vi "Comments.Add Wiring Description.vi"(8 "error in (no error)":errorcluster, 11 "Control Experiment in":refnum<class "Control Experiment.lvclass">) -> (0 "error out":errorcluster, 2 "Wiring Description":string, 3 "Control Experiment out":refnum<class "Control Experiment.lvclass">)   [LabVIEW 2019, in "Control Experiment.lvclass"]
uses:
  Control Experiment.lvclass
  Control Experiment.lvclass/Control Experiment.ctl
  <userlib>/LevyLab/Krohn Hite 7008/Instrument.KH7008.lvclass/Instrument.KH7008.ctl
  <userlib>/LevyLab/PLYM/YAML.lvclass
  <userlib>/LevyLab/Krohn Hite 7008/Instrument.KH7008.lvclass
panel:
  out "Numeric":i32
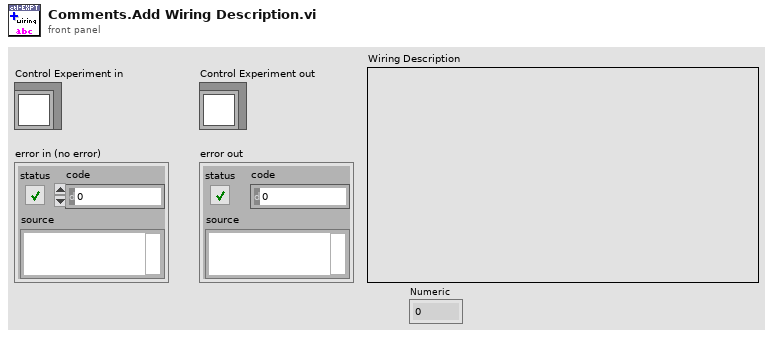
[diagram p1: front panel]
types:
  T1 = typedef "Instrument.KH7008.lvclass/SetAll-Array.ctl" = T2[]
  T2 = typedef "Instrument.KH7008.lvclass/SetAll-Cluster.ctl" = cluster{"Channel":T3, "Gain":T4, "Bandwidth Filter":T5, "Shunt Resistor":T6, "Coupling":T7, "Input Config":T8}
  T3 = typedef "Instrument.KH7008.lvclass/Channel-Enum.ctl" = enum16{"Channel 1", "Channel 2", "Channel 3", "Channel 4", "Channel 5", "Channel 6", "Channel 7", "Channel 8"}
  T4 = typedef "Instrument.KH7008.lvclass/Gain-Enum.ctl" = enum16{"1x", "10x", "100x", "1000x"}
  T5 = typedef "Instrument.KH7008.lvclass/Filter-Enum.ctl" = enum16{"OFF", "ON"}
  T6 = typedef "Instrument.KH7008.lvclass/Shunt-Enum.ctl" = enum16{"Open", "50 Ohms", "500 Ohms", "5k Ohms", "50k Ohms", "10M Ohm"}
  T7 = typedef "Instrument.KH7008.lvclass/Coupling-Enum.ctl" = enum16{"AC", "DC"}
  T8 = typedef "Instrument.KH7008.lvclass/Input Configuration-Enum.ctl" = enum16{"Ground", "SE+ (-gnd)", "SE- (+gnd)", "Differential"}
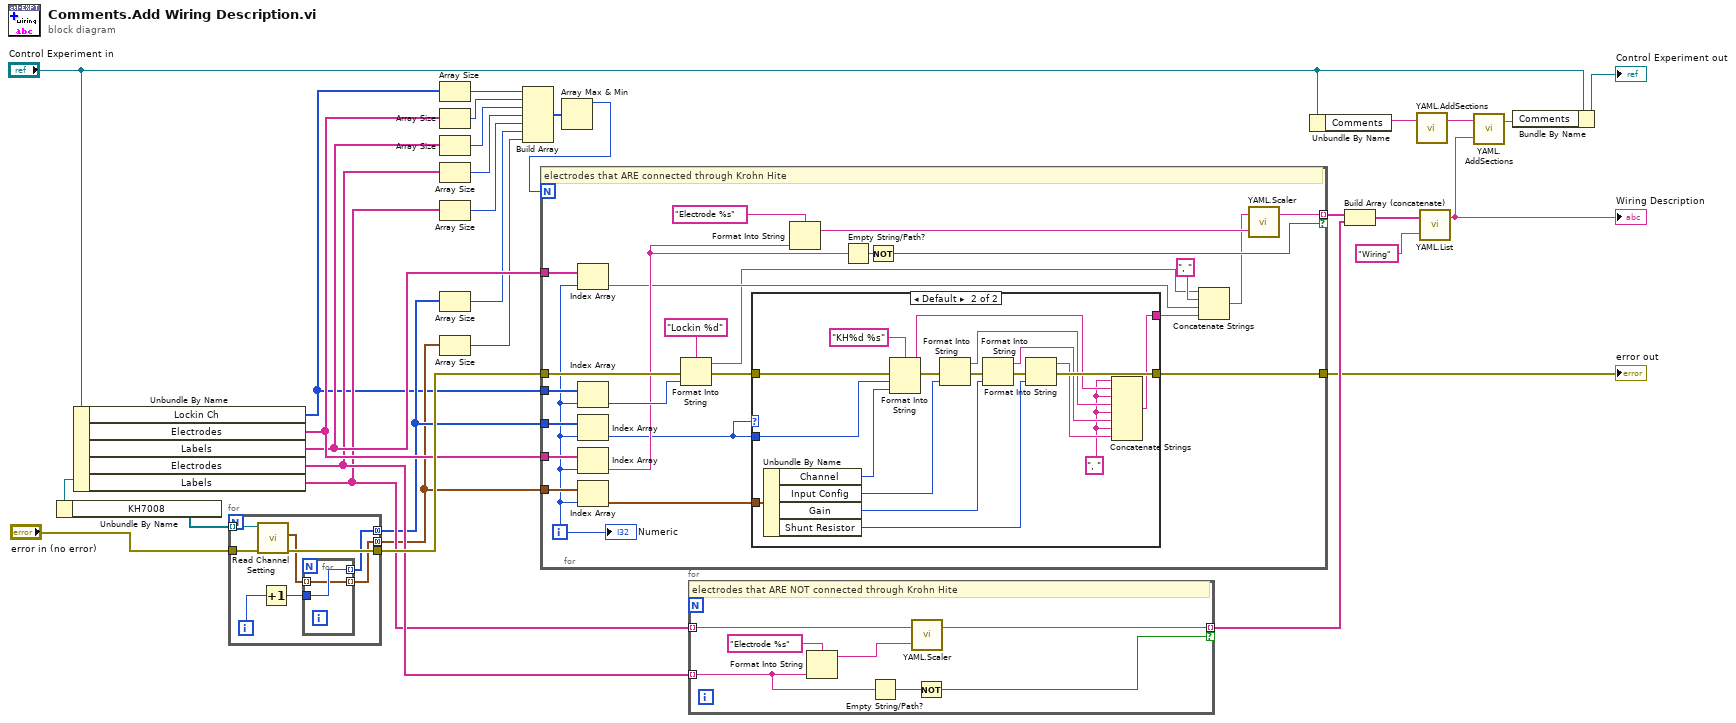
[diagram p0: block diagram]
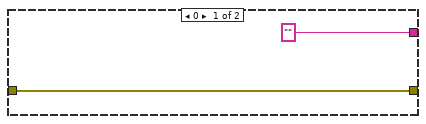
[diagram p2: hidden frame]
diagram:
  n1 = Unbundle By Name("Control Experiment in") -> ("KH7008"=w21:refnum<class "Instrument.KH7008.lvclass">[])
  n2 = Unbundle By Name("Control Experiment in") -> ("Lockin Ch"=w7:i32[], "Electrodes"=w16:string[], "Labels"=w15:string[], "Electrodes"=w14:string[], "Labels"=w13:string[])
  n3 = for {
    tunnel: [w32] -> w11 mode=concatenating
    tunnel: w21 -> [w37] mode=indexing
    tunnel: "error in (no error)" -> [w36]
    tunnel: [w38] -> w22
    tunnel: [w31] -> w12 mode=concatenating
    i -> [w35]
    n4 = call <userlib>:"Read Channel Setting.vi"("error in (no error)"=w36, "Instrument.KH7008 in"=w37) -> ("error out"=w38:errorcluster, "Channel Setting"=w33:T1)  [unwired: 7 in, 1 out]
    n5 = Increment(x=w35) -> (x+1=w34:i32)
    n6 = for {
      tunnel: w34 -> [w40]
      tunnel: w33 -> [w39] mode=indexing
      tunnel: [w40] -> w31 mode=indexing
      tunnel: [w39] -> w32 mode=indexing
    }
  }
  n7 = Array Size(array=w7) -> (size(s)=w10:i32)
  n8 = Array Size(array=w16) -> (size(s)=w9:i32)
  n9 = Array Size(array=w15) -> (size(s)=w8:i32)
  n10 = Array Size(array=w14) -> (size(s)=w6:i32)
  n11 = Array Size(array=w13) -> (size(s)=w5:i32)
  n12 = Array Size(array=w12) -> (size(s)=w4:i32)
  n13 = Array Size(array=w11) -> (size(s)=w3:i32)
  n14 = Build Array(w10, w9, w8, w6, w5, w4, w3) -> (w2:i32[])
  n15 = Array Max & Min(array=w2) -> (max value=w1:i32)  [unwired: 3 out]
  n16 = for {
    N: w1 -> [_]
    tunnel: w7 -> [w52]
    tunnel: w16 -> [w59]
    tunnel: w15 -> [w51]
    tunnel: [w56] -> w24 mode=indexing if=w62
    tunnel: w22 -> [w58]
    tunnel: [w54] -> w20
    tunnel: w11 -> [w61]
    tunnel: w12 -> [w53]
    i -> [w41]
    # "electrodes that ARE connected through Krohn Hite"
    n17 = Index Array(array=w51, index=w41) -> (element=w43:string)
    n18 = Index Array(array=w52, index=w41) -> (element=w50:i32)
    n19 = Index Array(array=w53, index=w41) -> (element=w45:i32)
    n20 = Index Array(array=w59, index=w41) -> (element=w49:string)
    n21 = Index Array(array=w61, index=w41) -> (element=w48:T2)
    n22 = Format Into String(format string="Lockin %d", error in=w58, w50) -> (resulting string=w42:string, error out=w64:errorcluster)  [unwired: 1 in]
    n23 = case shown="Default" w45 {
      tunnel: w64 -> [w66 w81]
      tunnel: ["" w67] -> w44
      tunnel: [w66 w75] -> w54
      tunnel: w45 -> [_ w74]
      tunnel: w48 -> [_ w73]
      frame 0 {
      }
      frame Default {
        w68 = ", "
        n24 = Unbundle By Name(w73) -> ("Channel"=w76:T3, "Input Config"=w80:T8, "Gain"=w79:T4, "Shunt Resistor"=w78:T6)
        n25 = Format Into String(format string="KH%d %s", error in=w81, w74, w76) -> (resulting string=w69:string, error out=w84:errorcluster)  [unwired: 1 in]
        n26 = Format Into String(error in=w84, w80) -> (resulting string=w70:string, error out=w83:errorcluster)  [unwired: 2 in]
        n27 = Format Into String(error in=w83, w79) -> (resulting string=w71:string, error out=w82:errorcluster)  [unwired: 2 in]
        n28 = Format Into String(error in=w82, w78) -> (resulting string=w72:string, error out=w75:errorcluster)  [unwired: 2 in]
        n29 = Concatenate Strings(w68, w69, w68, w70, w68, w71, w68, w72) -> (w67:string)
      }
    }
    n30 = Format Into String(format string="Electrode %s", w49) -> (resulting string=w57:string)  [unwired: 2 in, 1 out]
    n31 = Empty String/Path?(string/path=w49) -> (empty?=w63:bool)
    n32 = Not(x=w63) -> (.not. x?=w62:bool)
    n33 = Concatenate Strings(w42, ", ", w43, w44) -> (w47:string)
    n34 = call <userlib>:"YAML.Scaler.vi"("Key"=w57, "Scaler"=w47) -> ("Output"=w56:string)  [unwired: 1 in]
    "Numeric" <- w41
  }
  "error out" <- w20
  n35 = for {
    tunnel: [w85] -> w25 mode=indexing if=w89
    tunnel: w13 -> [w86] mode=indexing
    tunnel: w14 -> [w91] mode=indexing
    # "electrodes that ARE NOT connected through Krohn Hite"
    n36 = Format Into String(format string="Electrode %s", w91) -> (resulting string=w87:string)  [unwired: 2 in, 1 out]
    n37 = Empty String/Path?(string/path=w91) -> (empty?=w90:bool)
    n38 = call <userlib>:"YAML.Scaler.vi"("Key"=w87, "Scaler"=w86) -> ("Output"=w85:string)  [unwired: 1 in]
    n39 = Not(x=w90) -> (.not. x?=w89:bool)
  }
  n40 = Unbundle By Name("Control Experiment in") -> ("Comments"=w27:string)
  n41 = Build Array (concatenate)(w24, w25) -> (w26:string[])
  n42 = call <userlib>:"YAML.AddSections.vi"("Section 1"=w27) -> ("Output"=w29:string)  [unwired: 2 in]
  n43 = call <userlib>:"YAML.List.vi"("Key"="Wiring" ("string"), "lines"=w26) -> ("Output"=w17:string)  [unwired: 1 in]
  "Wiring Description" <- w17
  n44 = call <userlib>:"YAML.AddSections.vi"("Section 2"=w17, "Section 1"=w29) -> ("Output"=w30:string)  [unwired: 1 in]
  n45 = Bundle By Name(cluster="Control Experiment in", "Comments"=w30) -> (→"Control Experiment out":refnum<class "Control Experiment.lvclass">)
